vi "SCDP - Simeltaeneous Tx Rx Test.vi"() -> ()   [LabVIEW 2020]
uses:
  Typedefs/SDCP - Serial Port Control - Commands.ctl
  Typedefs/SDCP SMF logger - SMF with timestamp.ctl
  Typedefs/SDCP - Standard Message Frame Parameters - FGV - commands.ctl
panel:
  out "Elapsed time (ms)":u32
  out "Table updated":bool
  in  "Receive Table":i32(listbox)
  out "Number of elements \nin queue":i32
  in  "Parameter file path":path
  out "Number of remaining elements":i32
  out "Number of queued elements":i32
  in  "stop":bool
  in  "COM Port":refnum<visa-resource-name>
  in  "Baud rate":u32=9600
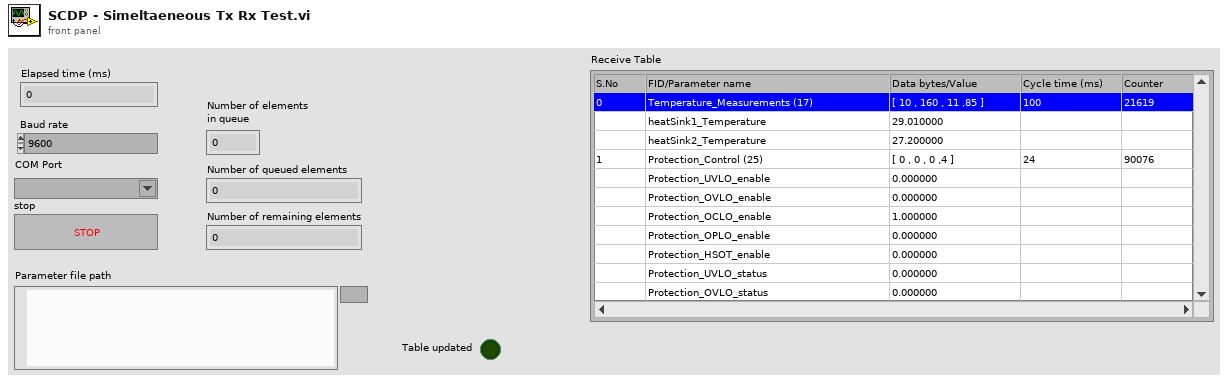
[diagram p1: front panel]
types:
  T1 = typedef "SDCP SMF logger - SMF with timestamp.ctl" = cluster{"Bytes":u8[], "Checksum":bool, "Time (ms)":u32, "Tx/Rx":string}
  T2 = typedef "SDCP - Standard Message Frame Parameters - FGV - commands.ctl" = enum16{"Write descriptors", "Read descriptors", "Read values", "Load parameters from file", "Write values"}
  T3 = typedef "SDCP - Serial Port Control - Commands.ctl" = enum16{"Open", "Read", "Write", "Get instance", "Close"}
  T4 = typedef "SDCP - SMF parameter descriptors.ctl" = cluster{"Frame name":string, "Frame ID":i32, "Data type":string, "Start Position":i32, "Length":i32, "Factor":dbl, "Offset":dbl, "Parameter name":string, "Value":string}
  T5 = typedef "SDCP - Log Table - Element.ctl" = cluster{"Data frame":u8[], "Cycle time (ms)":i32, "Count":i32, "Frame ID":i32, "Frame name":string, "Parameter names":string[], "Parameter values":string[]}
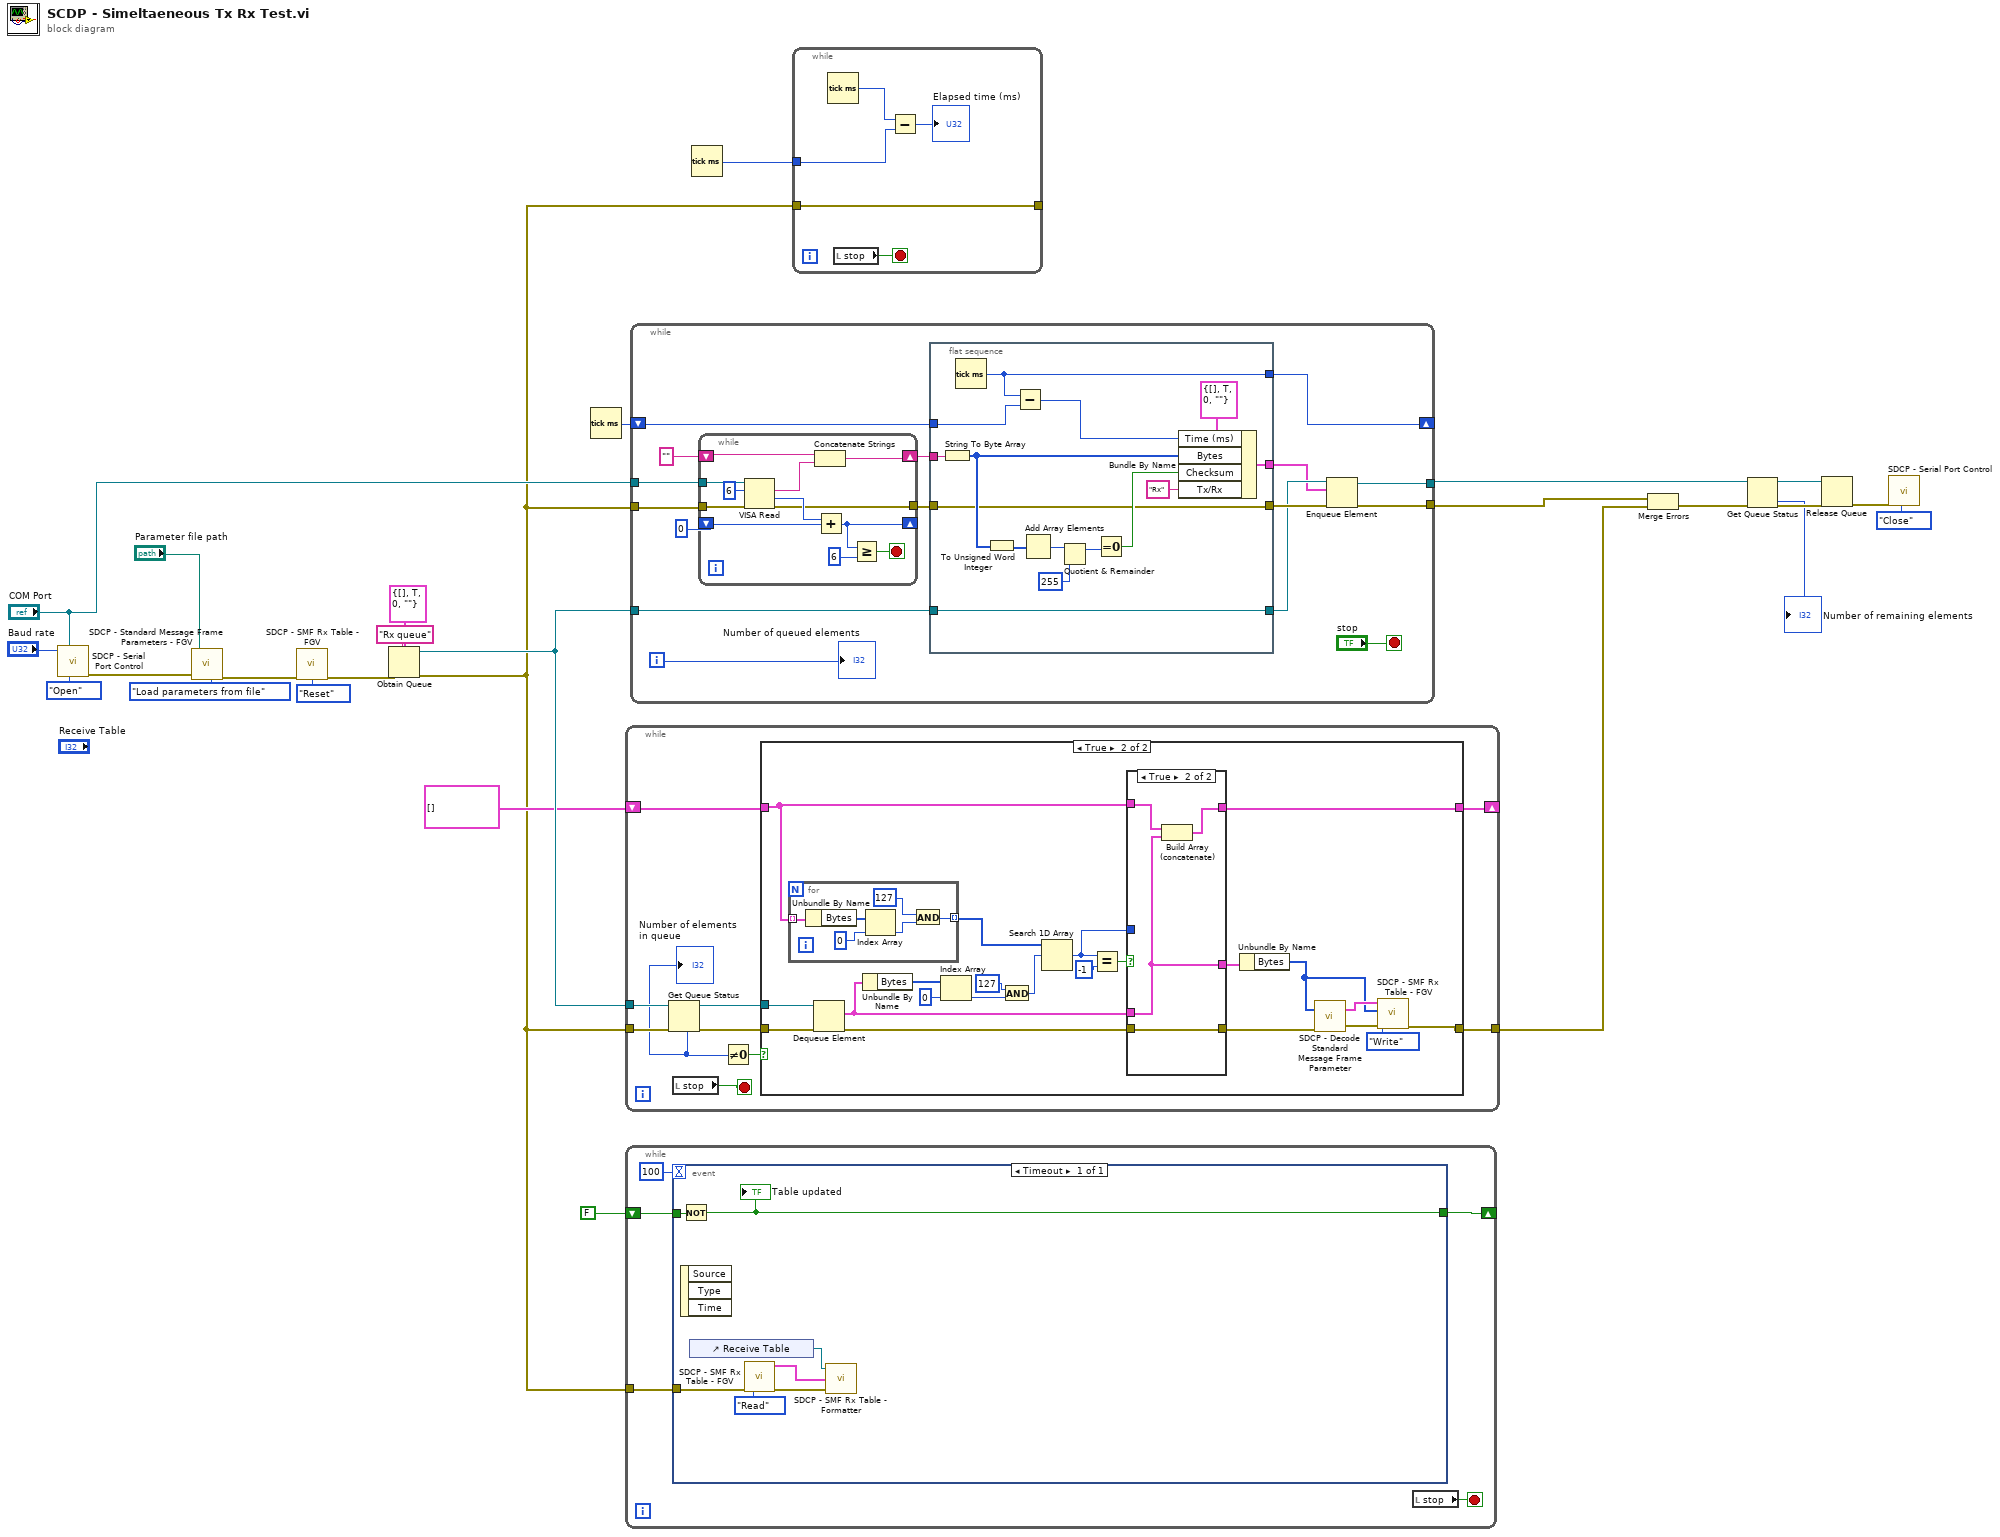
[diagram p0: block diagram]
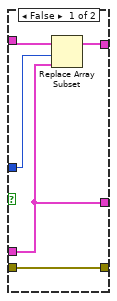
[diagram p3: hidden frame]
diagram:
  n1 = call "SDCP - Serial Port Control.vi"("Command"=SDCP_-_Serial_Port_Control_-_Commands."Open", "VISA resource name"="COM Port", "Baud rate"="Baud rate") -> ("error out"=w12:errorcluster)  [unwired: 6 in, 2 out]
  n2 = call "SDCP - Standard Message Frame Parameters - FGV.vi"("Parameter file path"="Parameter file path", "error in (no error)"=w12, "Command"=SDCP_-_Standard_Message_Frame_Parameters_-_FGV_-_commands."Load parameters from file") -> ("error out"=w8:errorcluster)  [unwired: 4 in, 1 out]
  n3 = call "SDCP - SMF Rx Table - FGV.vi"("error in (no error)"=w8, "Command"=enum16{"Reset", "Write", "Read"}."Reset") -> ("error out"=w7:errorcluster)  [unwired: 8 in, 1 out]
  n4 = Obtain Queue(name (unnamed)="Rx queue", element data type=T1 {"Bytes"=[], "Checksum"=TRUE, "Time (ms)"=0, "Tx/Rx"=""} ("SMF with timestamp"), error in (no error)=w7) -> (queue out=w10:refnum<queue>, error out=w2:errorcluster)  [unwired: 2 in, 1 out]
  n5 = Tick Count (ms)() -> (millisecond timer value=w21:u32)
  n6 = while {
    tunnel: w2 -> [w36]
    tunnel: w10 -> [w35]
    tunnel: [w31] -> w5
    shift-right: [w28] -> _
    shift-left: T1[] [] -> [w29]
    stop <- w30 stop-if-true
    n7 = Get Queue Status(queue=w35, error in (no error)=w36) -> (queue out=w32:refnum<queue>, error out=w33:errorcluster, # elements in queue=w27:i32)  [unwired: 1 in, 5 out]
    "Number of elements \nin queue" <- w27
    n8 = local read "stop"() -> (w30:bool)
    n9 = Not Equal To 0?(x=w27) -> (x != 0?=w34:bool)
    n10 = case shown="True" w34 {
      tunnel: w33 -> [w38 w60]
      tunnel: [w38 w42] -> w31
      tunnel: w32 -> [_ w59]
      tunnel: w29 -> [w37 w48]
      tunnel: [w37 w46] -> w28
      frame False {
      }
      frame True {
        n11 = for {
          tunnel: w48 -> [w75] mode=indexing
          tunnel: [w70] -> w54 mode=indexing
          n12 = Unbundle By Name(w75) -> ("Bytes"=w73:u8[])
          n13 = Index Array(array=w73, index=0) -> (element=w71:u8)
          n14 = And(x=u8 127, y=w71) -> (x .and. y?=w70:u8)
        }
        n15 = Dequeue Element(queue=w59, error in (no error)=w60) -> (element=w47:T1, error out=w51:errorcluster)  [unwired: 1 in, 2 out]
        n16 = Unbundle By Name(w47) -> ("Bytes"=w58:u8[])
        n17 = Index Array(array=w58, index=0) -> (element=w56:u8)
        n18 = And(x=u8 127, y=w56) -> (x .and. y?=w53:u8)
        n19 = Search 1D Array(1D array=w54, element=w53) -> (index of element=w49:i32)  [unwired: 1 in]
        n20 = Equal?(x=w49, y=-1) -> (x = y?=w50:bool)
        n21 = case shown="True" w50 {
          tunnel: w51 -> [w61 w68]
          tunnel: w49 -> [w63 _]
          tunnel: w48 -> [w65 w69]
          tunnel: w47 -> [w62 w67]
          tunnel: [w64 w66] -> w46
          tunnel: [w61 w68] -> w45
          tunnel: [w62 w67] -> w44
          frame False {
            n22 = Replace Array Subset(array=w65, new element=w62, index=w63) -> (w64:T1[])
          }
          frame True {
            n23 = Build Array (concatenate)(w69, w67) -> (w66:T1[])
          }
        }
        n24 = Unbundle By Name(w44) -> ("Bytes"=w40:u8[])
        n25 = call "SDCP - Decode Standard Message Frame Parameter.vi"("error in (no error)"=w45, "Bytes in"=w40) -> ("error out"=w43:errorcluster, "SMF Parameters out"=w41:T4[])
        n26 = call "SDCP - SMF Rx Table - FGV.vi"("error in (no error)"=w43, "Command"=enum16{"Reset", "Write", "Read"}."Write", "Bytes in"=w40, "Parameter descriptors"=w41) -> ("error out"=w42:errorcluster)  [unwired: 6 in, 1 out]
      }
    }
  }
  n27 = while {
    tunnel: w2 -> [w79]
    shift-right: [w76] -> _
    shift-left: FALSE -> [w77]
    stop <- w80 stop-if-true
    n28 = event shown="[0] Timeout" {
      selector: _ -> [_]
      dyn-events: _ -> [_]
      timeout: 100 -> [_]
      tunnel: w79 -> [w85]
      tunnel: w77 -> [w87]
      tunnel: [w86] -> w76
      event Timeout {
        n29 = Not(x=w87) -> (.not. x?=w86:bool)
        "Table updated" <- w86
        n30 = event-data() -> ()  [unwired: 1 in, 3 out]
        n31 = control-ref of="Receive Table"() -> (w81:refnum<vi>)
        n32 = call "SDCP - SMF Rx Table - FGV.vi"("error in (no error)"=w85, "Command"=enum16{"Reset", "Write", "Read"}."Read") -> ("error out"=w83:errorcluster, "Elements of log table"=w82:T5[])  [unwired: 8 in]
        n33 = call "SDCP - SMF Rx Table - Formatter.vi"("error in (no error)"=w83, "Elements of table"=w82, "Table reference"=w81) -> ()  [unwired: 2 in, 1 out]
      }
    }
    n34 = local read "stop"() -> (w80:bool)
  }
  n35 = while {
    tunnel: w2 -> [w103]
    tunnel: "COM Port" -> [w101]
    tunnel: w10 -> [w96]
    tunnel: [w92] -> w18
    tunnel: [w90] -> w17
    shift-right: [w88] -> _
    shift-left: w21 -> [w98]
    i -> [w89]
    stop <- "stop" stop-if-true
    n36 = while {
      tunnel: w103 -> [w130]
      shift-right: [w120] -> w99
      shift-left: "" -> [w121]
      tunnel: w101 -> [w129]
      shift-right: [w124] -> _
      shift-left: 0 -> [w126]
      tunnel: [w122] -> w97
      stop <- w125 stop-if-true
      n37 = VISA Read(VISA resource name=w129, byte count=u32 6, error in (no error)=w130) -> (read buffer=w119:string, return count=w127:u32, error out=w122:errorcluster)  [unwired: 1 out]
      n38 = Concatenate Strings(w121, w119) -> (w120:string)
      n39 = Add(x=w127, y=w126) -> (x+y=w124:u32)
      n40 = Greater Or Equal?(x=w124, y=u32 6) -> (x >= y?=w125:bool)
    }
    n41 = flat-sequence {
      tunnel: w99 -> [w118]
      tunnel: w98 -> [w109]
      tunnel: [w108] -> w93
      tunnel: w97 -> [w107]
      tunnel: [w107] -> w95
      tunnel: w96 -> [w106]
      tunnel: [w106] -> w94
      tunnel: [w104] -> w88
      frame #0 {
        n42 = String To Byte Array(string=w118) -> (unsigned byte array=w116:u8[])
        n43 = Tick Count (ms)() -> (millisecond timer value=w104:u32)
        n44 = To Unsigned Word Integer(number=w116) -> (unsigned 16bit integer=w115:u16[])
        n45 = Subtract(x=w104, y=w109) -> (x-y=w105:u32)
        n46 = Add Array Elements(numeric array=w115) -> (sum=w114:u16)
        n47 = Quotient & Remainder(x=w114, y=u16 255) -> (x-y*floor(x/y)=w112:u16)  [unwired: 1 out]
        n48 = Equal To 0?(x=w112) -> (x = 0?=w111:bool)
        n49 = Bundle By Name(cluster=T1 {"Bytes"=[], "Checksum"=TRUE, "Time (ms)"=0, "Tx/Rx"=""} ("SMF with timestamp"), "Time (ms)"=w105, "Bytes"=w116, "Checksum"=w111, "Tx/Rx"="Rx") -> (w108:T1)
      }
    }
    n50 = Enqueue Element(queue=w94, element=w93, error in (no error)=w95) -> (queue out=w90:refnum<queue>, error out=w92:errorcluster)  [unwired: 1 in, 1 out]
    "Number of queued elements" <- w89
  }
  n51 = Tick Count (ms)() -> (millisecond timer value=w1:u32)
  n52 = while {
    tunnel: w2 -> [w132]
    tunnel: w1 -> [w133]
    tunnel: [w132] -> _
    stop <- w135 stop-if-true
    n53 = Tick Count (ms)() -> (millisecond timer value=w134:u32)
    n54 = local read "stop"() -> (w135:bool)
    n55 = Subtract(x=w134, y=w133) -> (x-y=→"Elapsed time (ms)":u32)
  }
  n56 = Merge Errors(w18, w5) -> (w6:errorcluster)
  n57 = Get Queue Status(queue=w17, error in (no error)=w6) -> (queue out=w15:refnum<queue>, error out=w16:errorcluster, # elements in queue=→"Number of remaining elements":i32)  [unwired: 1 in, 5 out]
  n58 = Release Queue(queue=w15, error in (no error)=w16) -> (error out=w20:errorcluster)  [unwired: 1 in, 2 out]
  n59 = call "SDCP - Serial Port Control.vi"("Command"=SDCP_-_Serial_Port_Control_-_Commands."Close", "error in (no error)"=w20) -> ()  [unwired: 7 in, 3 out]
